vi "SaveDataFile.vi"(4 "Arrays format":string, 5 "Humidity":dbl, 6 "Array Titles":string, 7 "Temperature":dbl, 8 "Error In":errorcluster, 9 "Actual array lengths":i32, 10 "no. of arrays":i32, 11 "Data Array":dbl[][](array[numeric])) -> (0 "Error Out":errorcluster, 1 "Path + Filename OUT":string, 2 "Pathname OUT":string, 3 "Filename OUT":string)   [LabVIEW 2013]
uses:
  globals/QC_RunInformation.vi
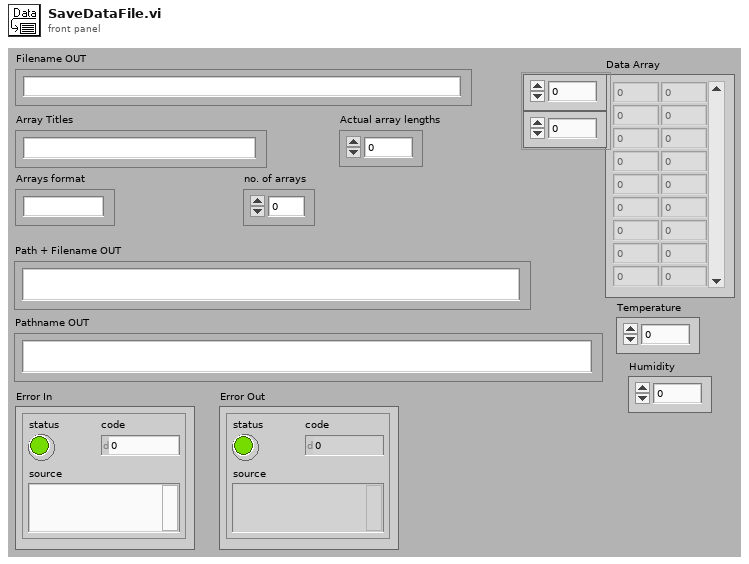
[diagram p1: front panel]
types:
  T1 = enum16{"open", "open or create", "create or replace", "create"}
  T2 = cluster{"Sensor Serial No.:":string, "Wafer Serial No.:":string, "Batch:":string, "Manufacturer:":string, "Device Category:":string, "Database Serial No.:":string, "Initiated:":string, "Test":string, "Instruments used:":string, "Probeplan used:":string, "End of Run comment:":string, "User:":string}
  T3 = cluster{"Institute":string, "Manufacturers":string[], "Devices":string[], "Serialnumbers Lookup DB":string, "Data directory":string, "www directory":string, "List of known users":string[]}
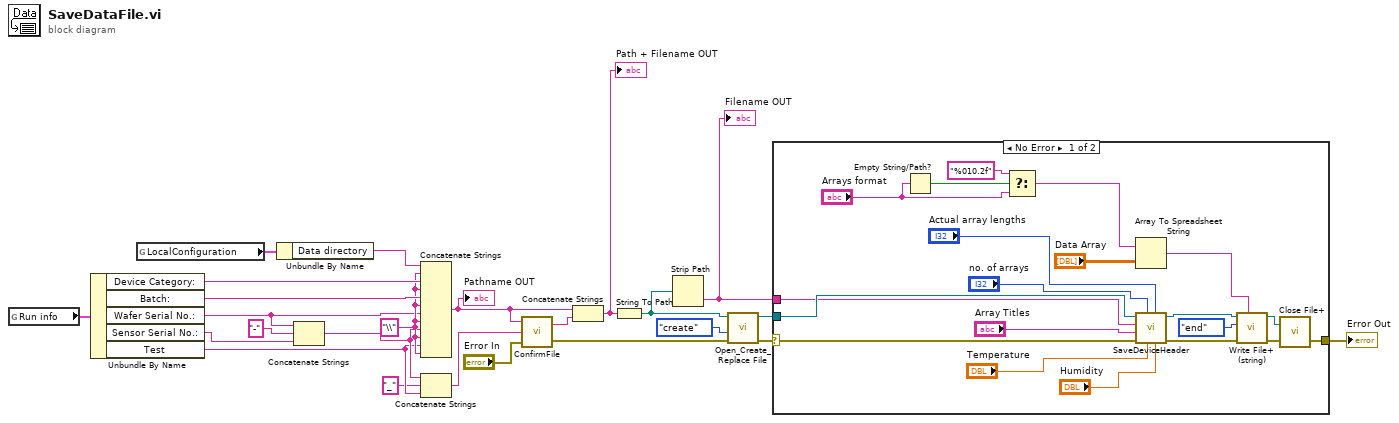
[diagram p0: block diagram]
diagram:
  w14 = "\\"
  n1 = global read "QC_RunInformation.vi" "Run info"() -> (w23:T2)
  n2 = Unbundle By Name(w23) -> ("Device Category:"=w21:string, "Batch:"=w20:string, "Wafer Serial No.:"=w12:string, "Sensor Serial No.:"=w11:string, "Test"=w8:string)
  n3 = global read "QC_RunInformation.vi" "LocalConfiguration"() -> (w24:T3)
  n4 = Unbundle By Name(w24) -> ("Data directory"=w22:string)
  n5 = Concatenate Strings(w12, "-", w11) -> (w10:string)
  n6 = Concatenate Strings(w22, w14, w21, w14, w20, w14, w12, w14, w10, w14, w8, w14) -> (w3:string)
  "Pathname OUT" <- w3
  n7 = Concatenate Strings(w10, "_", w8) -> (w9:string)
  n8 = call "ConfirmFile.vi"("Error In"="Error In", "Filename IN"=w9, "Pathname IN"=w3) -> ("Error Out"=w4:errorcluster, "Filename:"=w2:string)
  n9 = Concatenate Strings(w3, w2) -> (w1:string)
  "Path + Filename OUT" <- w1
  n10 = String To Path(string=w1) -> (path=w16:path)
  n11 = Strip Path(path=w16) -> (name=w17:string)  [unwired: 1 out]
  "Filename OUT" <- w17
  n12 = call <vilib>:"Open_Create_Replace File.vi"("error in (no error)"=w4, "function (open:0)"=T1."create", "file path"=w16) -> ("error out"=w15:errorcluster, "refnum"=w18:refnum<file>)  [unwired: 5 in, 2 out]
  n13 = case shown="No Error" w15 {
    selector: w15 -> [w44 w45]
    tunnel: w18 -> [w32 _]
    tunnel: w17 -> [w31 _]
    tunnel: [w27 w45] -> w6
    frame No Error {
      n14 = Empty String/Path?(string/path="Arrays format") -> (empty?=w41:bool)
      n15 = Select(t="%010.2f", s=w41, f="Arrays format") -> (s? t:f=w39:string)
      n16 = Array To Spreadsheet String(array="Data Array", 3:w39) -> (spreadsheet string=w38:string)  [unwired: 1 in]
      n17 = call "SaveDeviceHeader.vi"("Humidity"="Humidity", "Array Lengths"="Actual array lengths", "Temperature"="Temperature", "no. of arrays"="no. of arrays", "error in (no error)"=w44, "Array Titles"="Array Titles", "Filename"=w31, "File Refnum in"=w32) -> ("error out"=w34:errorcluster, "File Refnum out"=w33:refnum<file>)  [unwired: 1 in, 1 out]
      n18 = call <vilib>:"Write File+ (string).vi"("string"=w38, "error in (no error)"=w34, "pos mode (rel. to end:1)"=enum16{"start", "end", "current"}."end", "refnum"=w33) -> ("error out"=w37:errorcluster, "dup refnum"=w35:refnum<file>)  [unwired: 3 in, 1 out]
      n19 = call <vilib>:"Close File+.vi"("error in (no error)"=w37, "refnum"=w35) -> ("error out"=w27:errorcluster)  [unwired: 3 in, 2 out]
    }
    frame Error {
    }
  }
  "Error Out" <- w6
